vi "JSONRPC-SplitArray.vi"(7 "unquote strings (false)":bool, 11 "input string":string) -> (3 "array":string[](array[string]))   [LabVIEW 2019]
doc: "Searches for a JSON array in <b>input string</b> and creates an array with the elements found."
panel:
  # "SplitArray"
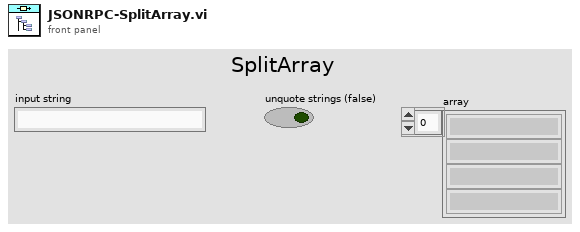
[diagram p1: front panel]
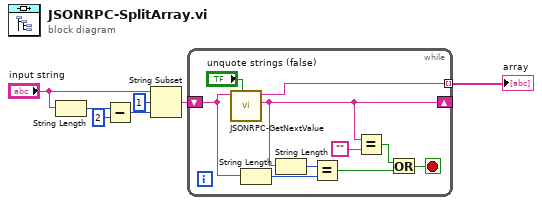
[diagram p0: block diagram]
diagram:
  n1 = String Length(string="input string") -> (length=w3:i32)
  n2 = Subtract(x=w3, y=2) -> (x-y=w1:i32)
  n3 = String Subset(string="input string", offset (0)=1, length (rest)=w1) -> (substring=w5:string)
  n4 = while {
    shift-right: [w8] -> _
    shift-left: w5 -> [w12]
    tunnel: [w17] -> w7 mode=indexing
    stop <- w13 stop-if-true
    n5 = call "JSONRPC-GetNextValue.vi"("unquote strings (false)"="unquote strings (false)", "input string"=w12) -> ("after"=w8:string, "next"=w17:string)  [unwired: 8 in]
    n6 = String Length(string=w12) -> (length=w15:i32)
    n7 = String Length(string=w8) -> (length=w14:i32)
    n8 = Equal?(x=w14, y=w15) -> (x = y?=w10:bool)
    n9 = Equal?(x=w8, y="") -> (x = y?=w9:bool)
    n10 = Or(x=w9, y=w10) -> (x .or. y?=w13:bool)
  }
  "array" <- w7
